vi "prima_apl_v1.vi"() -> ()   [LabVIEW 2009]
panel:
  out "Dispozitiv de afisare":string caption="Caption \"Dispozitiv de afisare\""
  # "Prima aplicatie realizata in LabView"
  # "Aplicatia afiseaza un mesaj de bun venit in momentul cand este lansata"
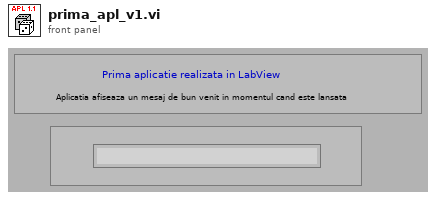
[diagram p1: front panel]
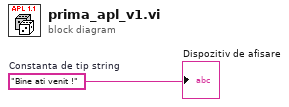
[diagram p0: block diagram]
diagram:
  w1 = "Bine ati venit !"  # Constanta de tip string
  "Dispozitiv de afisare" <- w1
